vi "Panel Wrapper.vi"(10 "Actor":refnum<class "Actor.lvclass">, 11 "Panel in":refnum<class "Panel.lvclass">) -> ()   [LabVIEW 2021, in "Panel.lvclass"]
uses:
  Panel.lvclass
  <vilib>/jettl/jettl/jettl/Actor/Actor.lvclass
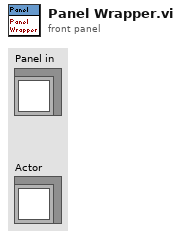
[diagram p1: front panel]
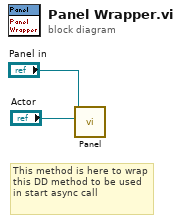
[diagram p0: block diagram]
diagram:
  # "This method is here to wrap this DD method to be used in start async call"
  n1 = call-dynamic "Panel.vi"("Actor"="Actor", "Panel"="Panel in") -> ()  [unwired: 10 in]
